vi "WT1600(Init).vi"(0 "VISA session 2":refnum<visa-resource-name>, 7 "ID Query (T: Check)":bool=TRUE, 9 "Reset (T: Reset)":bool=TRUE, 11 "error in (no error)":errorcluster) -> (4 "VISA session":refnum<visa-resource-name>, 15 "error out":errorcluster)   [LabVIEW 2016]
doc: "This VI passes the addressing information in the instrument descriptor to the Instr Open VI and returns the instrument ID. You can optionally reset the instrument by setting the front panel reset control. You must run this VI before using any of the instrument driver VIs for this instrument.\n\nNote : All parameters of ASRLx interface are stored to the \"visaconf.ini\" file. To configure serial interface use please T&M Explorer or Measurement & Automation Explorer."
panel:
  # "Note : All parameters of ASRLx interface are stored \nto the \"visaconf.ini\" file. To configure serial interface \nuse please \"T&M Explorer\" or \"Measurement & \nAutomation Explorer\"."
  # "Check\nDon't Check"
  # "Reset\nDon't Reset"
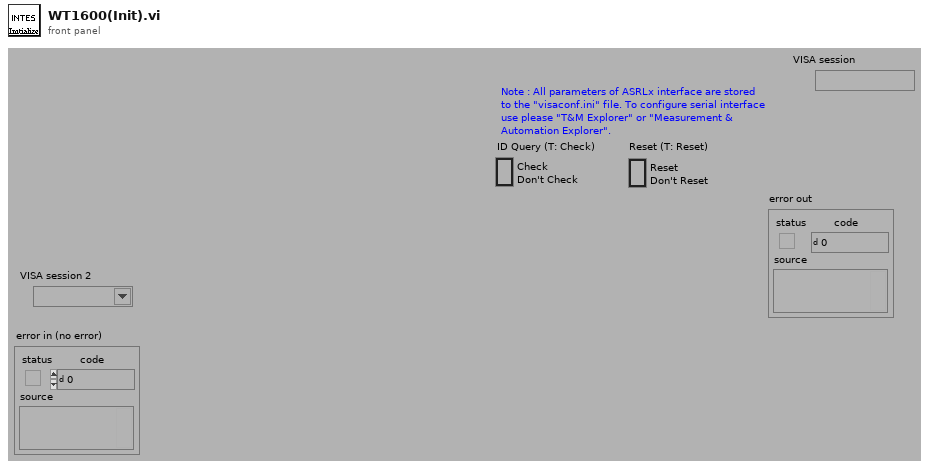
[diagram p1: front panel]
types:
  T1 = cluster{"status":bool, "code":i32, "VI name":string}
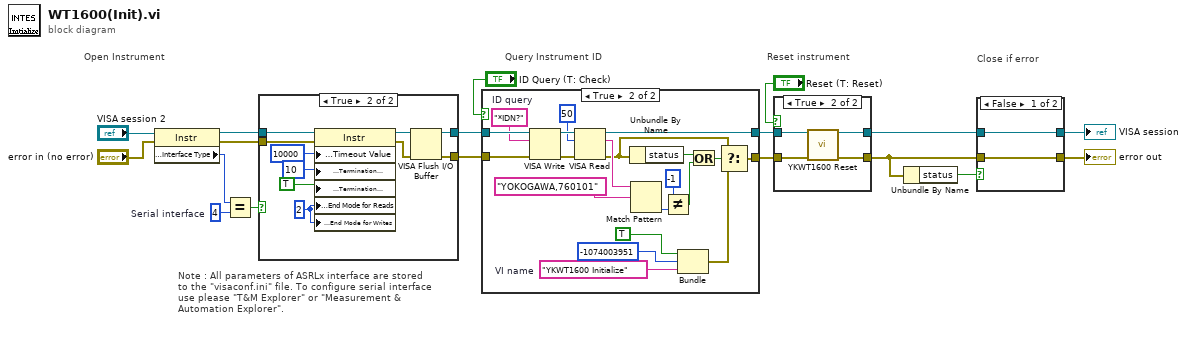
[diagram p0: block diagram]
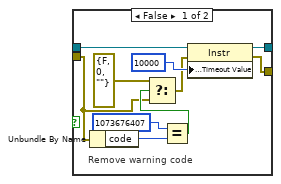
[diagram p2: hidden frame]
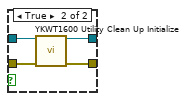
[diagram p3: hidden frame]
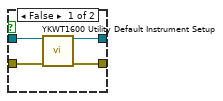
[diagram p4: hidden frame]
diagram:
  w3 = u16 4  # Serial interface
  # "Note : All parameters of ASRLx interface are stored \nto the \"visaconf.ini\" file. To configure serial interface \nuse please \"T&M Explorer\" or \"Measurement & \nAutomation Explorer\"."
  # "Close if error"
  # "Query Instrument ID"
  # "Reset instrument"
  # "Open Instrument"
  n1 = property class="Instr"(reference="VISA session 2", error in="error in (no error)") -> (reference out=w7:refnum<visa-resource-name>, error out=w6:errorcluster, "Interface Information:Interface Type"=w4:u16)
  n2 = Equal?(x=w4, y=w3) -> (x = y?=w5:bool)
  n3 = case shown="True" w5 {
    tunnel: [w28 w30] -> w9
    tunnel: [w27 w29] -> w8
    tunnel: w7 -> [w26 w34]
    tunnel: w6 -> [w21 w33]
    frame False {
      # "Remove warning code"
      n4 = Unbundle By Name(w21) -> ("code"=w24:i32)
      n5 = Equal?(x=1073676407, y=w24) -> (x = y?=w22:bool)
      n6 = Select(t=errorcluster {"status"=FALSE, "code"=0, "source"=""}, s=w22, f=w21) -> (s? t:f=w19:errorcluster)
      n7 = property class="Instr"(reference=w26, error in=w19, "General Settings:Timeout Value"=u32 10000 ("Tmo Value")) -> (reference out=w28:refnum<visa-resource-name>, error out=w27:errorcluster)
    }
    frame True {
      w35 = u16 2
      n8 = property class="Instr"(reference=w34, error in=w33, "General Settings:Timeout Value"=u32 10000 ("Tmo Value"), "Message Based Settings:Termination Character"=u8 10, "Message Based Settings:Termination Character Enable"=TRUE, "Serial Settings:End Mode for Reads"=w35, "Serial Settings:End Mode for Writes"=w35) -> (reference out=w32:refnum<visa-resource-name>, error out=w31:errorcluster)
      n9 = VISA Flush I/O Buffer(VISA resource name=w32, error in (no error)=w31) -> (VISA resource name out=w30:refnum<visa-resource-name>, error out=w29:errorcluster)  [unwired: 1 out]
    }
  }
  n10 = case shown="True" "ID Query (T: Check)" {
    tunnel: [w39 w58] -> w17
    tunnel: [w40 w56] -> w18
    tunnel: w9 -> [w40 w54]
    tunnel: w8 -> [w39 w53]
    frame False {
    }
    frame True {
      w48 = "YKWT1600 Initialize"  # VI name
      w52 = "*IDN?"  # ID query
      n11 = VISA Write(VISA resource name=w54, write buffer=w52, error in (no error)=w53) -> (VISA resource name out=w55:refnum<visa-resource-name>, error out=w60:errorcluster)  [unwired: 1 out]
      n12 = VISA Read(VISA resource name=w55, byte count=u32 50, error in (no error)=w60) -> (VISA resource name out=w56:refnum<visa-resource-name>, read buffer=w46:string, error out=w42:errorcluster)  [unwired: 1 out]
      n13 = Unbundle By Name(w42) -> ("status"=w41:bool)
      n14 = Match Pattern(string=w46, regular expression="YOKOGAWA,760101") -> (offset past match=w50:i32)  [unwired: 4 out]
      n15 = Not Equal?(x=-1, y=w50) -> (x != y?=w43:bool)
      n16 = Bundle(TRUE, -1074003951, "VI name"=w48) -> (w57:cluster{bool, i32, "VI name":string})  [unwired: 1 out]
      n17 = Or(x=w41, y=w43) -> (x .or. y?=w44:bool)
      n18 = Select(t=w42, s=w44, f=w57) -> (s? t:f=w58:T1)
    }
  }
  n19 = case shown="True" "Reset (T: Reset)" {
    tunnel: w17 -> [w63 w68]
    tunnel: [w64 w67] -> w11
    tunnel: w18 -> [w62 w65]
    tunnel: [w61 w66] -> w14
    frame False {
      n20 = call "YKWT1600 Utility Default Instrument Setup"("VISA session"=w62, "error in (no error)"=w63) -> ("dup VISA session"=w61:refnum<visa-resource-name>, "error out"=w64:errorcluster)  [unwired: 12 out]
    }
    frame True {
      n21 = call "YKWT1600 Reset.vi"("VISA session"=w65, "error in (no error)"=w68) -> ("dup VISA session"=w66:refnum<visa-resource-name>, "error out"=w67:errorcluster)  [unwired: 12 out]
    }
  }
  n22 = Unbundle By Name(w11) -> ("status"=w10:bool)
  n23 = case shown="False" w10 {
    tunnel: w11 -> [w69 w74]
    tunnel: w14 -> [w70 w73]
    tunnel: [w70 w72] -> w13
    tunnel: [w69 w71] -> w12
    frame False {
    }
    frame True {
      n24 = call "YKWT1600 Utility Clean Up Initialize"("VISA session"=w73, "error in (no error)"=w74) -> ("dup VISA session"=w72:refnum<visa-resource-name>, "error out"=w71:errorcluster)  [unwired: 12 out]
    }
  }
  "VISA session" <- w13
  "error out" <- w12
